vi "Write ItemsList.vi"(8 "error in (no error)":errorcluster, 10 "Items List":string[](array[string]), 11 "Msg_Error.lvclass in":refnum<class "ListSelection.lvclass">) -> (0 "error out":errorcluster, 3 "Msg_Error.lvclass out":refnum<class "ListSelection.lvclass">)   [LabVIEW 2012, in "ListSelection.lvlib" / "ListSelection.lvclass"]
uses:
  ListSelection.lvclass
  ListSelection.lvclass/ListSelection.ctl
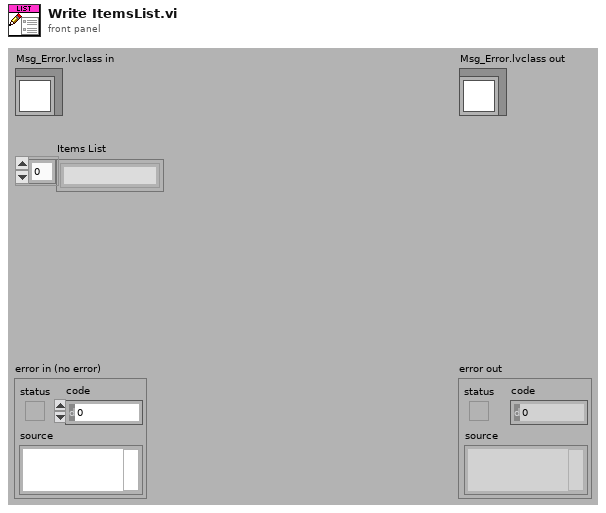
[diagram p1: front panel]
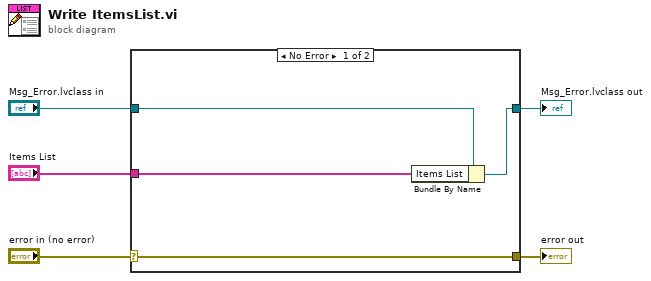
[diagram p0: block diagram]
diagram:
  n1 = case shown="No Error" "error in (no error)" {
    selector: "error in (no error)" -> [w9 w10]
    tunnel: [w9 w10] -> w4
    tunnel: [w7 w11] -> w2
    tunnel: "Msg_Error.lvclass in" -> [w8 w11]
    tunnel: "Items List" -> [w6 _]
    frame No Error {
      n2 = Bundle By Name(cluster=w8, "Items List"=w6) -> (w7:refnum<class "ListSelection.lvclass">)
    }
    frame Error {
    }
  }
  "error out" <- w4
  "Msg_Error.lvclass out" <- w2
